vi "Process.vi"(8 "error in":errorcluster, 11 "Edit.Funnel":refnum<class "Edit.Funnel.lvclass">) -> (0 "error out":errorcluster, 3 "Edit.Funnel out":refnum<class "Edit.Funnel.lvclass">)   [LabVIEW 2019, in "Edit.Funnel.lvclass"]
doc: "---------------------------------------------------------------\nJKI State Machine Objects™\nhttp://jki.net/state-machine-objects/\nCopyright (C) 2005-2015, JKI <info@jki.net>\nALL RIGHTS RESERVED"
uses:
  Edit.Funnel.lvclass
  C:/Program Files (x86)/National Instruments/LabVIEW 2019/vi.lib/JKI/JKI SMO/SMO/SMO.lvclass
  <vilib>/JKI/JKI SMO/SMO/Typedefs/Parent Call--Enum.ctl
  Settings/Funnel Settings/Funnel Settings.lvclass/Funnel Settings.ctl
  Settings/ObjectSettings/ObjectSettings.lvclass/ObjectSettings.ctl
  subVIs/typedefs/Schedule Types/Schedule--Constant.ctl
  Settings/Setting Database/Setting Database.lvclass
  Settings/Funnel Settings/Funnel Settings.lvclass
  C:/Users/Albro/Documents/GitHub/AFM-Lithography/lvsrc/Classes/Settings/ObjectSettings/ObjectSettings.lvclass
  <vilib>/Utility/miscctls.llb/LVPointTypeDef.ctl
  <vilib>/JKI/JKI SMO/SMO/SMO.lvclass/SMO.ctl
  Settings/Setting Database/Typedefs/PrivateEvents--Setting Database.Copy Settings To Group.ctl
  Settings/Setting Database/Typedefs/PrivateEvents--Setting Database.SetDefaultFunnel.ctl
  Settings/Setting Database/Typedefs/PrivateEvents--Setting Database.CopyActiveFunnelToAll.ctl
  Settings/Funnel Settings/Accessors/Write Bottom Segments.vi
  Settings/ObjectSettings/Accessors/Write Resistance.vi
  Settings/ObjectSettings/Accessors/Read Speed Settings.vi
  Settings/ObjectSettings/Accessors/Read Voltage Settings.vi
  Settings/ObjectSettings/Accessors/Write Enabled.vi
  Settings/ObjectSettings/Accessors/Write Voltage Schedule.vi
  Settings/ObjectSettings/Accessors/Write Speed Schedule.vi
  Settings/ObjectSettings/Accessors/Write Direction.vi
  Settings/Funnel Settings/Accessors/Write Smooth Segments.vi
  Settings/ObjectSettings/Accessors/Read Enabled.vi
  Settings/ObjectSettings/Accessors/Read Direction.vi
  Settings/Funnel Settings/Accessors/Read Smooth Segments.vi
  Settings/Funnel Settings/Accessors/Read Bottom Segments.vi
  Settings/ObjectSettings/Accessors/Read Speed Schedule.vi
  Settings/ObjectSettings/Accessors/Read Voltage Schedule.vi
  Settings/ObjectSettings/Accessors/Read Resistance.vi
  <vilib>/JKI/JKI SMO/SMO/Private/ReftoDVR--SMO.vi
  Edit/Edit.lvclass
  <vilib>/JKI/JKI SMO/SMO/SMO.lvclass
  Settings/ObjectSettings/ObjectSettings.lvclass
panel:
  in  "Apply":bool
  in  "Apply All":bool
  out "Group String":string
  out "ID String":string
  in  "Copy to All":bool
  in  "Smooth Segments":dbl caption="Numeric 2"
  in  "Direction":u16(ring) caption="Ring" items=["Forward", "Backward"]
  in  "Speed Schedule":u16(ring) caption="Ring" items=["Constant", "Ramp", "Fn. Generator", "Formula"]
  in  "Voltage Schedule":u16(ring) caption="Ring" items=["Constant", "Ramp", "Fn. Generator", "Formula"]
  in  "Speed Settings":bool
  in  "Voltage Settings":bool
  in  "Enabled?":bool=TRUE
  in  "Voltage (V)":dbl caption="Numeric 2"
  in  "Speed (um/s)":dbl caption="Numeric 2"
  in  "Set Resistance":T1(ring) caption="Enum"
  in  "Bottom Segments":dbl caption="Numeric 2"
  in  "Save Default":bool
  # "For instructions on how to use the JKI State Machine Objects, examples and video tutorials, visit:\nhttp://jki.net/state-machine-objects/\n\nJKI State Machine Objects™\nhttp://jki.net/state-machine-objects/\nCopyright (C) 2005-2015, JKI <info@jki.net>\nALL RIGHTS RESERVED"
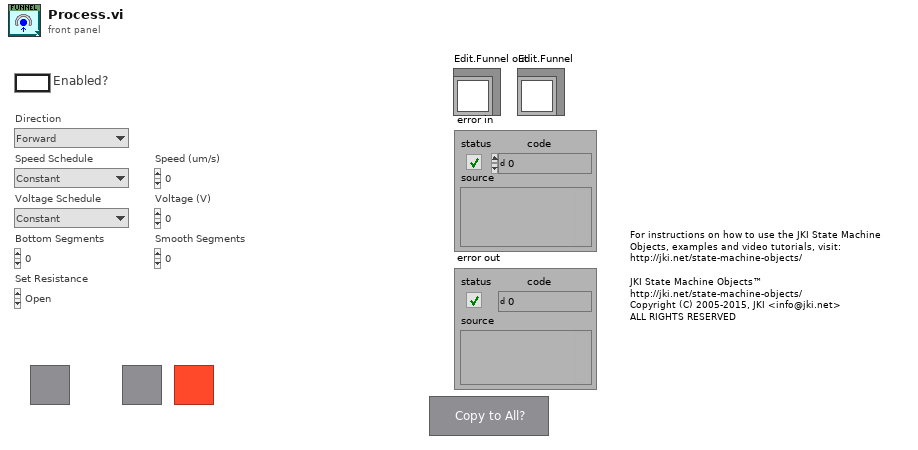
[diagram p1: front panel]
types:
  T1 = enum16{"Open", "Discharge Tip", "0 ohm", "100 kohm", "10 Mohm", "1 Gohm"}
  T2 = typedef "SMO.lvclass/Parent Call--Enum.ctl" = enum16{"Allows parent to run", "Does not request parent to run"}
  T3 = typedef "Schedule--Constant.ctl" = cluster{"Value":dbl}
  T4 = enum32{"invalid app kind", "Development System", "Run Time System", "Student Edition", "Embedded LabVIEW", "Evaluation", "Custom"}
  T5 = typedef "LVPointTypeDef.ctl" = cluster{"Horizontal":i16, "Vertical":i16}
  T6 = enum8{"Enabled", "Disabled", "Disabled and Grayed Out"}
  T7 = enum32{"Invalid", "Standard", "Closed", "Hidden", "Minimized", "Maximized"}
  T8 = enum32{"Bad", "Idle", "Run top level", "Running"}
  T9 = typedef "Setting Database.lvclass/PrivateEvents--Setting Database.Copy Settings To Group.ctl" = cluster{"Name":string, "Group":string}
  T10 = typedef "Setting Database.lvclass/PrivateEvents--Setting Database.SetDefaultFunnel.ctl" = bool
  T11 = typedef "Setting Database.lvclass/PrivateEvents--Setting Database.CopyActiveFunnelToAll.ctl" = bool
  T12 = typedef "Setting Database.lvclass/PublicEvents--Setting Database.NewActiveFunnel.ctl" = refnum<class "Funnel Settings.lvclass">
  T13 = cluster{"Core":cluster{"Current VI Reference":refnum<vi>, "Close Panel on Exit?":bool, "error":errorcluster}, "Self":refnum<class "Edit.Funnel.lvclass">, "SettingDB":refnum<class "Setting Database.lvclass">, "Funnel Settings":refnum<class "Funnel Settings.lvclass">}
  T14 = cluster{"Current VI Reference":refnum<vi>, "Close Panel on Exit?":bool, "error":errorcluster}
  T15 = enum16{"Always On", "Always Off", "Off While Running"}
  T16 = typedef "SMO.lvclass/Protected Events.ctl" = cluster{"StopProcesses":refnum<user-event>, "AbortProcesses":refnum<user-event>, "Config Changed":refnum<user-event>, "Dependency":refnum<user-event>}
  T17 = typedef "Setting Database.lvclass/PublicEvents--Cluster.ctl" = cluster{"NewActivePath":refnum<user-event>, "PathsUpdated":refnum<user-event>, "RectanglesUpdated":refnum<user-event>, "NewActiveRectangle":refnum<user-event>, "NewActiveFunnel":refnum<user-event>, "FunnelsUpdated":refnum<user-event>, "NewActiveDot":refnum<user-event>, "DotsUpdated":refnum<user-event>}
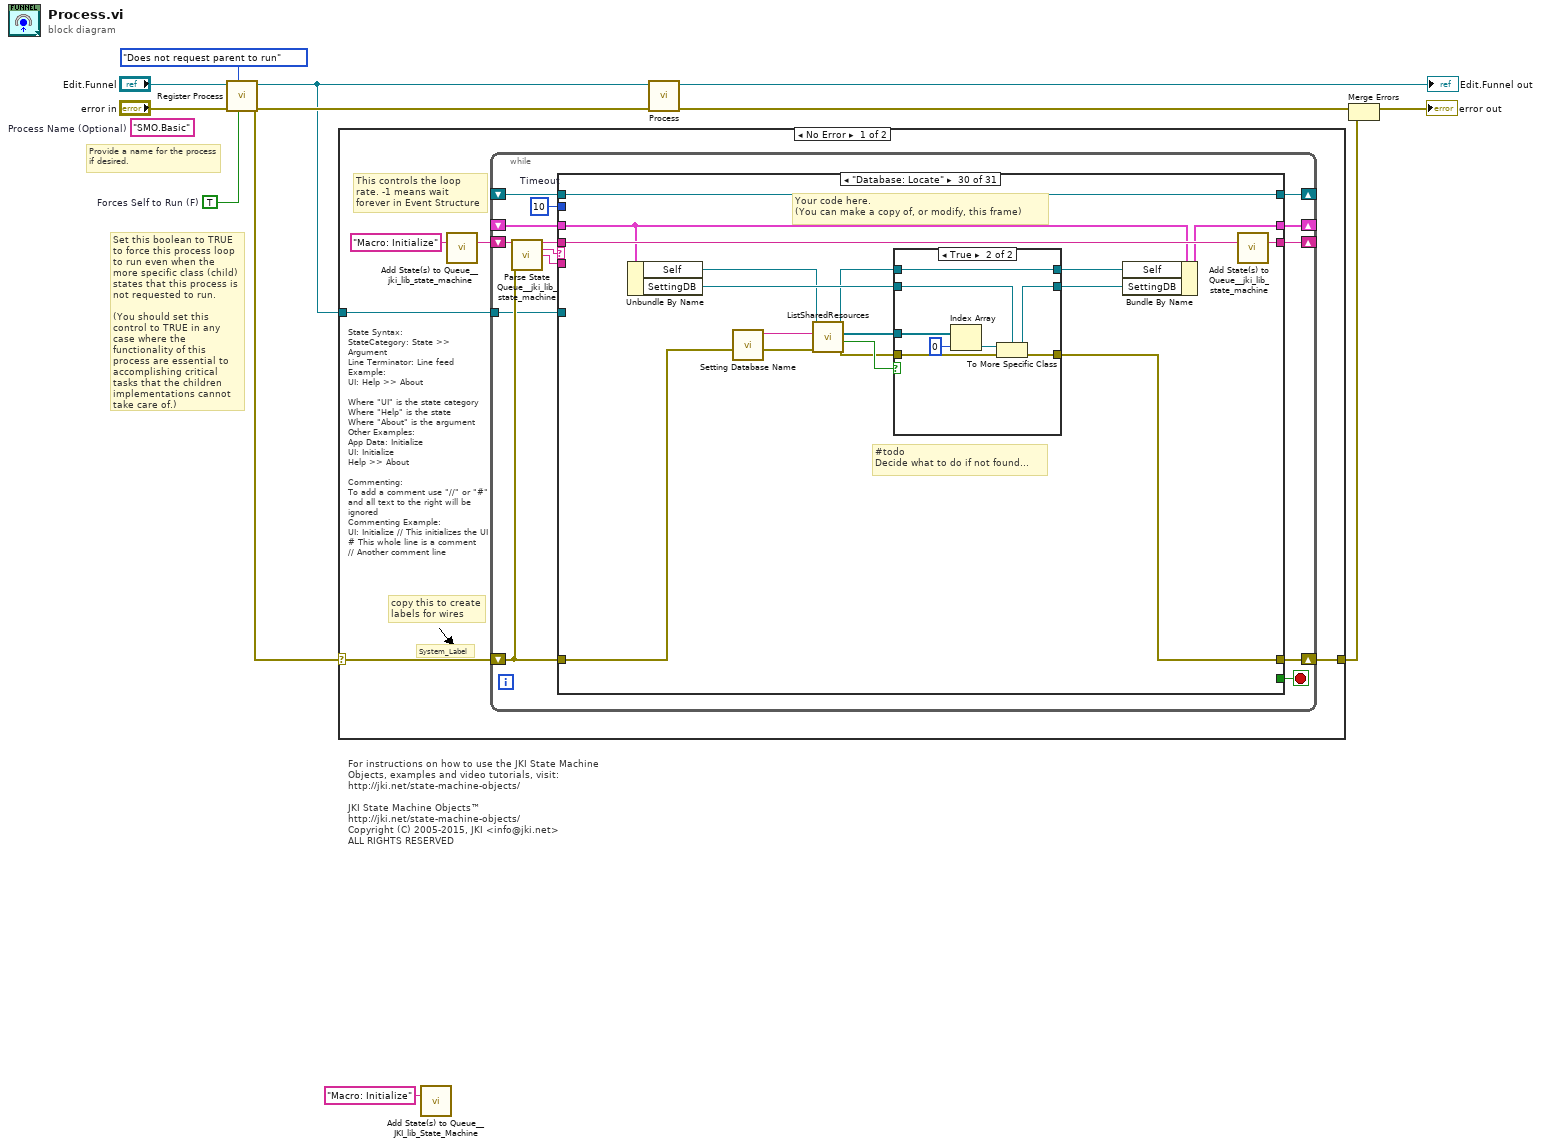
[diagram p0: block diagram]
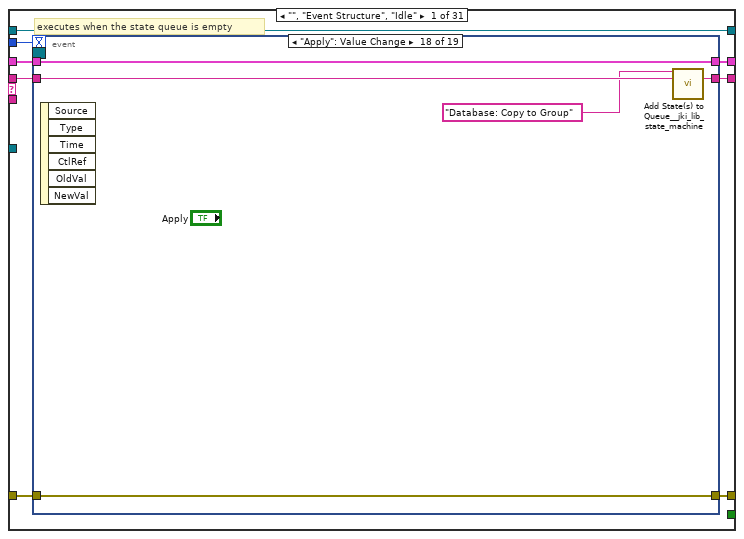
[diagram p2: hidden frame]
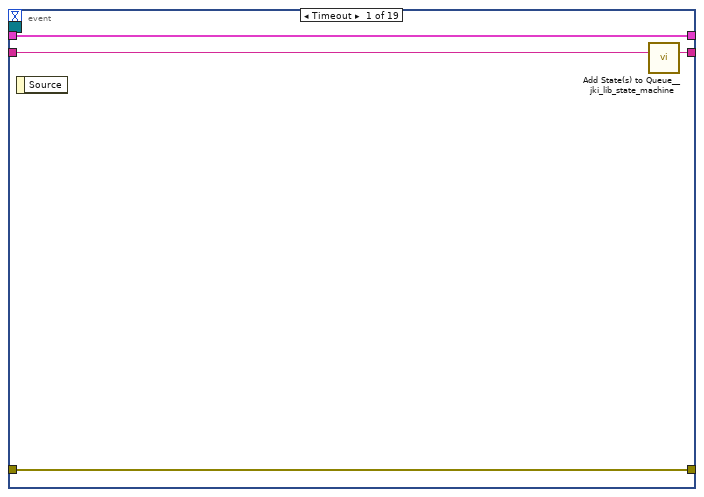
[diagram p3: hidden frame]
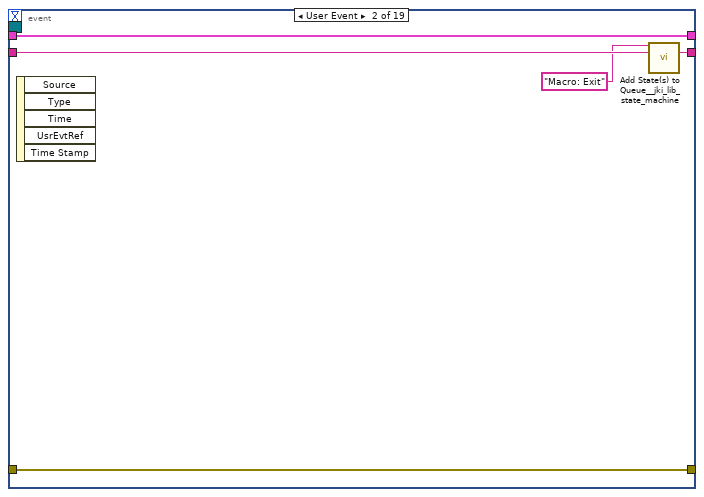
[diagram p4: hidden frame]
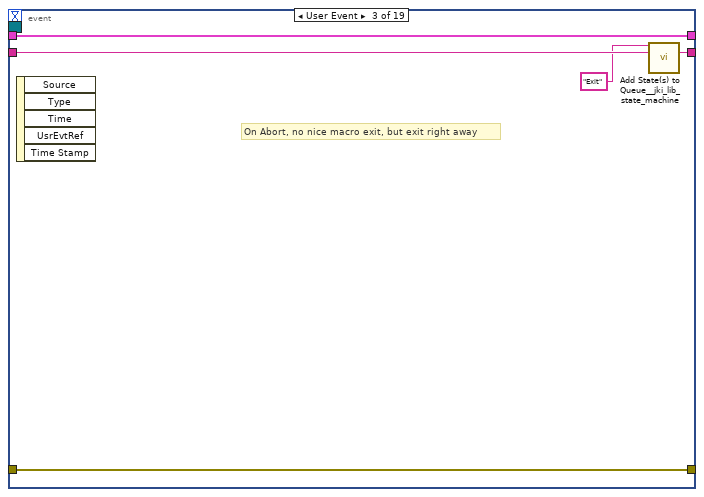
[diagram p5: hidden frame]
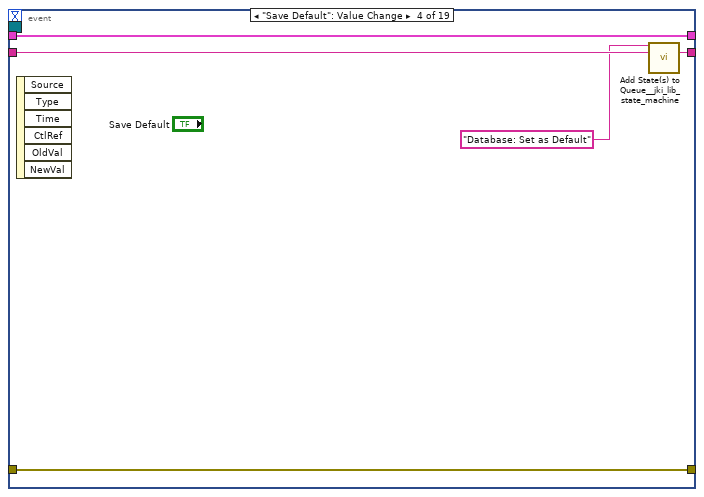
[diagram p6: hidden frame]
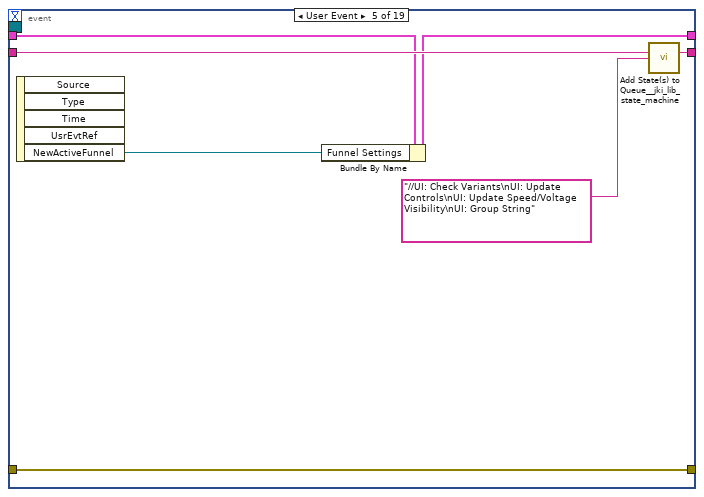
[diagram p7: hidden frame]
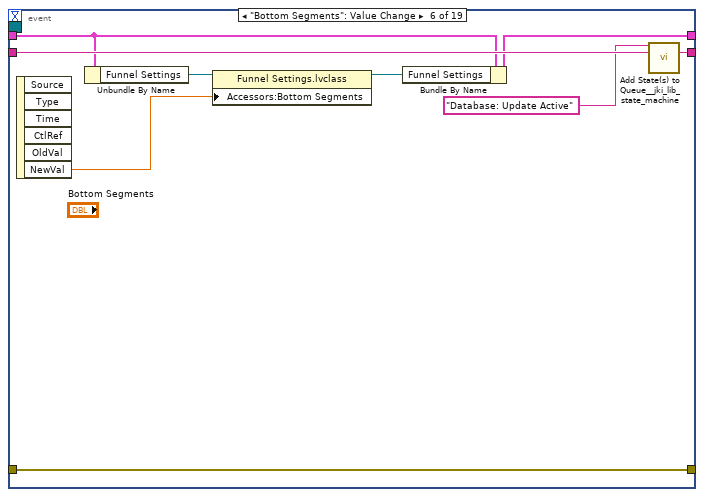
[diagram p8: hidden frame]
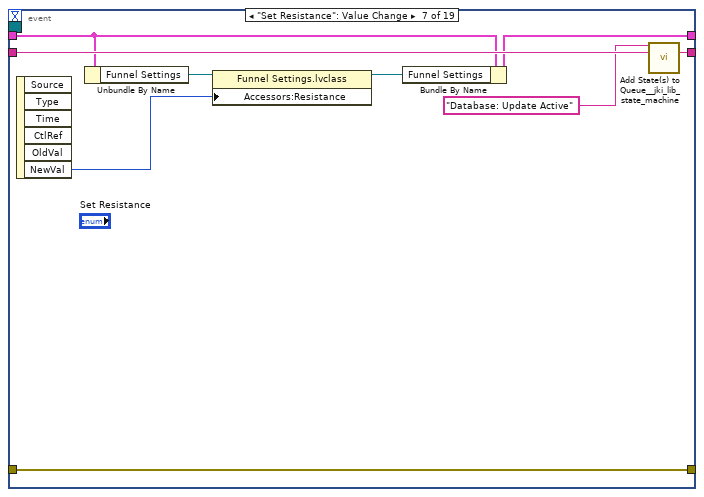
[diagram p9: hidden frame]
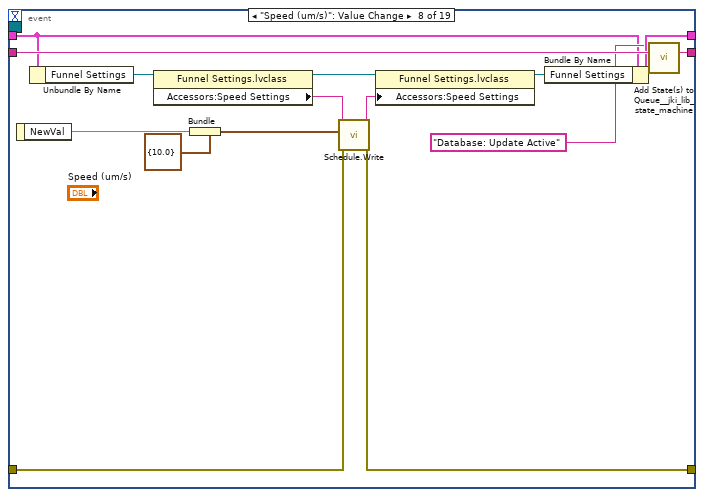
[diagram p10: hidden frame]
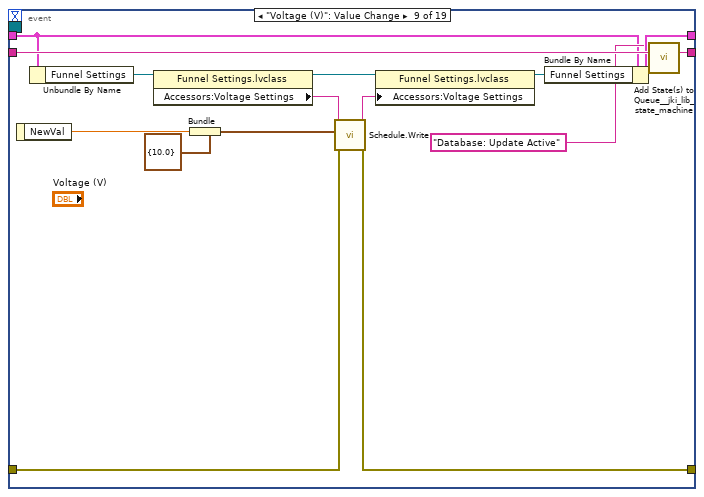
[diagram p11: hidden frame]
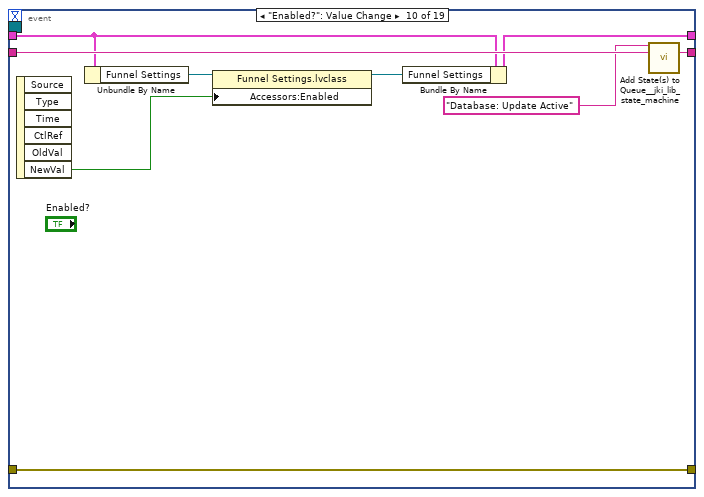
[diagram p12: hidden frame]
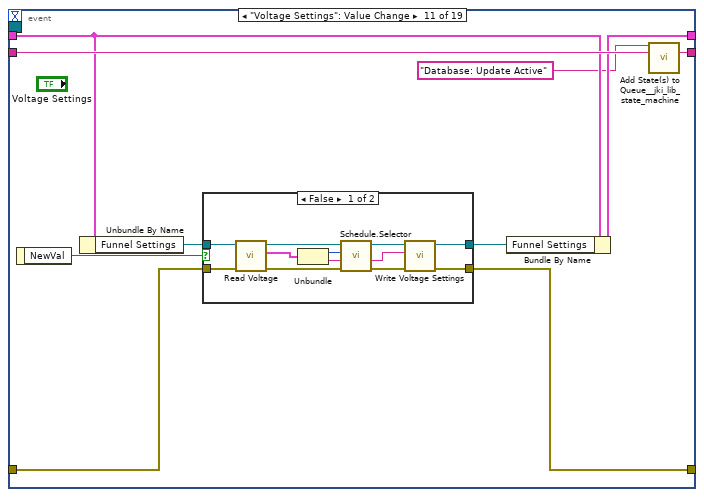
[diagram p13: hidden frame]
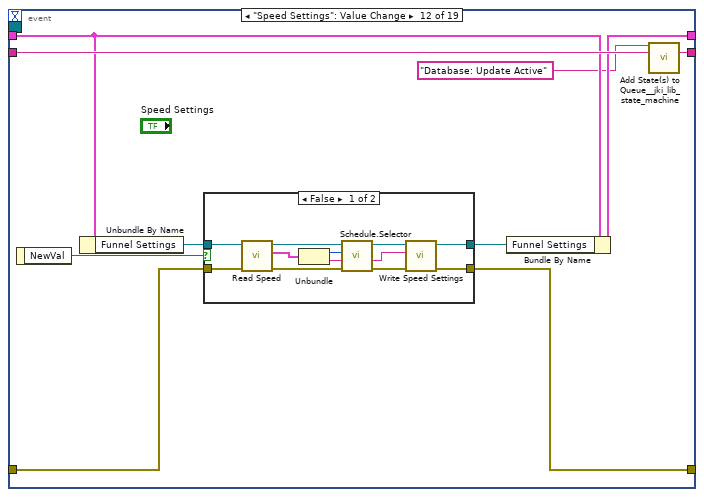
[diagram p15: hidden frame]
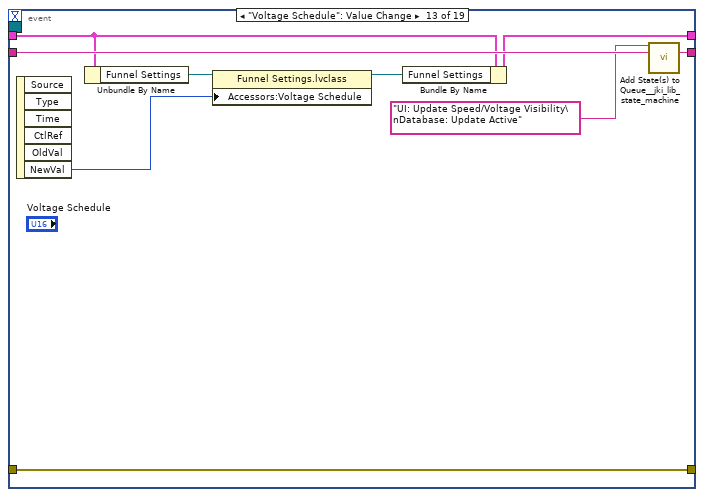
[diagram p17: hidden frame]
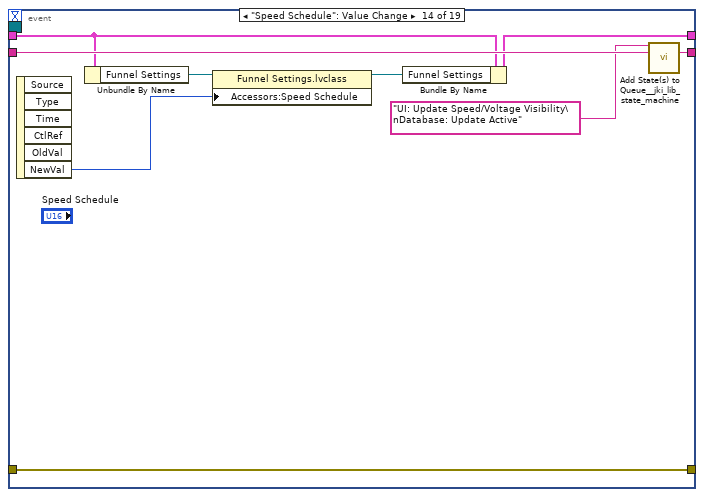
[diagram p18: hidden frame]
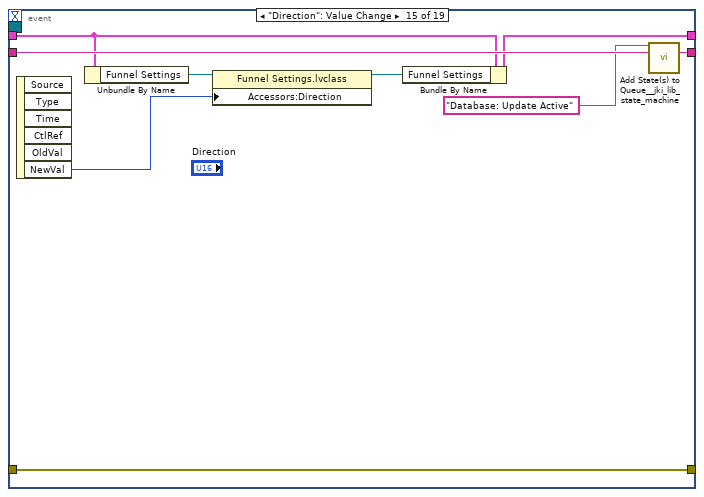
[diagram p19: hidden frame]
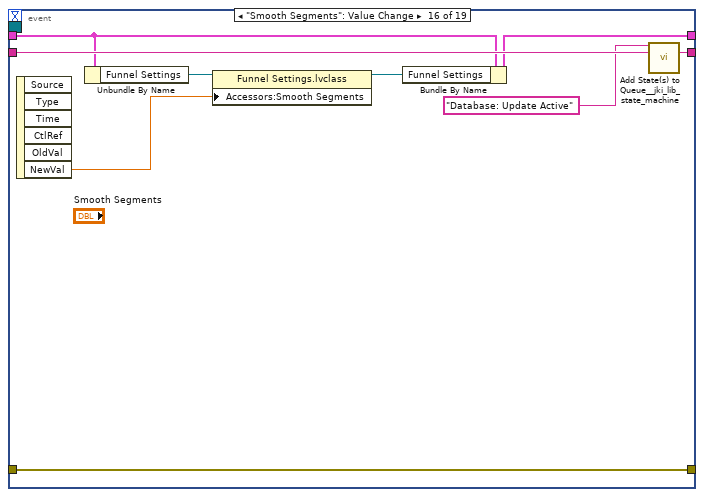
[diagram p20: hidden frame]
diagram:
  w3 = TRUE  # Forces Self to Run (F)
  (unwired) "SMO.Basic"  # Process Name (Optional)
  # "Provide a name for the process\nif desired."
  # "Set this boolean to TRUE to force this process loop to run even when the more specific class (child) states that this process is not requested to run.\n\n(You should set this control to TRUE in any case where the functionality of this process are essential to accomplishing critical tasks that the children implementations cannot take care of.)"
  # "For instructions on how to use the JKI State Machine Objects, examples and video tutorials, visit:\nhttp://jki.net/state-machine-objects/\n\nJKI State Machine Objects™\nhttp://jki.net/state-machine-objects/\nCopyright (C) 2005-2015, JKI <info@jki.net>\nALL RIGHTS RESERVED"
  n1 = call <vilib>:"Register Process.vi"("Forces Self to Run (F)"=w3, "Parent Call"=Parent_Call--Enum."Does not request parent to run", "error in (no error)"="error in", "SMO"="Edit.Funnel") -> ("error out"=w8:errorcluster, "SMO out"=w1:refnum<class "Edit.Funnel.lvclass">)  [unwired: 6 in]
  n2 = case shown="No Error" w8 {
    selector: w8 -> [w14 w583]
    tunnel: w1 -> [w13 _]
    tunnel: [w12 w583] -> w5
    frame No Error {
      # "State Syntax:\nStateCategory: State >> Argument\nLine Terminator: Line feed\nExample:\nUI: Help >> About\n\nWhere \"UI\" is the state category\nWhere \"Help\" is the state\nWhere \"About\" is the argument\nOther Examples:\nApp Data: Initialize\nUI: Initialize\nHelp >> About\n\nCommenting:\nTo add a comment use \"//\" or \"#\" and all text to the right will be ignored\nCommenting Example:\nUI: Initialize // This initializes the UI\n# This whole line is a comment\n// Another comment line"
      # "copy this to create labels for wires"
      # "This controls the loop rate. -1 means wait forever in Event Structure"
      # "System_Label"
      n3 = call <vilib>:"Add State(s) to Queue__jki_lib_state_machine.vi"("State(s) in (\"\")"="Macro: Initialize") -> ("States Out"=w15:string)  [unwired: 14 in]
      n4 = while "JKI - String-Based Queued State Machine (Basic) v1.0" {
        shift-right: [w23] -> _
        shift-left: _ -> [w22]
        shift-right: [w26] -> w12
        shift-left: w14 -> [w20]
        shift-right: [w25] -> _
        shift-left: w15 -> [w27]
        shift-right: [w19] -> _
        shift-left: _ -> [w18]
        tunnel: w13 -> [w17]
        stop <- w24 stop-if-true
        w21 = 10  # Timeout
        n5 = call <vilib>:"Parse State Queue__jki_lib_state_machine.vi"("State Queue"=w27, "Error In (no error)"=w20) -> ("Remaining States"=w29:string, "Current State"=w30:string, "Arguments"=w28:string)  [unwired: 11 in]
        n6 = case shown="\"Database: Locate\"" w30 {
          selector: w30 -> [_ _ w232 _ _ _ _ _ _ _ _ _ _ _ _ _ _ _ _ _ _ _ _ _ _ _ _ _ _ _ _]
          tunnel: w29 -> [w38 w226 w230 w251 w265 w271 w276 w288 w295 w300 w313 w327 w351 w366 w373 w392 w404 w436 w450 w464 w469 w480 w485 w498 w504 w509 w524 w534 w544 w561 w582]
          tunnel: w28 -> [_ _ _ _ _ _ _ _ _ _ _ _ _ _ w369 _ w399 _ _ _ _ _ _ _ _ _ _ _ _ _ _]
          tunnel: w22 -> [w36 w223 w231 w244 w252 w267 w273 _ w292 w297 w303 w320 w345 w358 w368 w390 w400 w433 w447 w451 w466 w473 w482 w494 w502 w506 w514 w526 w540 w548 w578]
          tunnel: [w35 w224 w235 w249 errorcluster {"status"=FALSE, "code"=0, "source"=""} ("error out") w266 w274 w280 w290 w298 w305 w322 w349 w363 w370 w379 w397 w434 w448 w462 w467 w471 w483 w493 w500 w507 w512 w529 w536 w546 w575] -> w26
          tunnel: w20 -> [w34 w224 w234 w249 w259 _ w274 w279 w291 w298 w307 w321 w349 w362 w371 w389 w398 w434 w448 w462 w467 w470 w483 w492 w500 w507 w511 w528 w537 w545 w574]
          tunnel: [w37 w225 w233 w250 w264 w270 w275 w287 w294 w299 w312 w326 w350 w365 w372 w391 w403 w435 w449 w463 w468 w479 w484 w497 w503 w508 w523 w533 w543 w560 w581] -> w25
          tunnel: [_ _ _ _ _ TRUE _ _ _ _ _ _ _ _ _ _ _ _ _ _ _ _ _ _ _ _ _ _ _ _ _] -> w24
          tunnel: [w33 w223 w231 w243 w258 w267 w273 w286 w292 w297 w303 w320 w345 w359 w368 w390 w400 w433 w447 w451 w466 w473 w482 w494 w502 w506 w515 w527 w541 w547 w579] -> w23
          tunnel: w21 -> [w32 _ _ _ _ _ _ _ _ _ _ _ _ _ _ _ _ _ _ _ _ _ _ _ _ _ _ _ _ _ _]
          tunnel: [w31 w222 w227 w239 w262 w268 w272 w284 w289 w296 w311 w325 w346 w361 w367 w378 w402 w432 w446 w461 w465 w478 w481 w496 w501 w505 w522 w532 w542 w559 w580] -> w19
          tunnel: w18 -> [w31 w222 w227 w239 w262 w268 w272 w284 w289 w296 w311 w325 w346 w361 w367 w378 w402 w432 w446 w461 w465 w478 w481 _ w501 w505 w522 w532 w542 w559 w580]
          tunnel: w17 -> [_ _ _ _ _ _ _ w282 _ _ _ _ _ _ _ _ _ _ _ _ _ _ _ _ _ _ _ _ _ _ _]
          frame "", "Event Structure", "Idle" {
            # "executes when the state queue is empty"
            n7 = event shown="[17] \"Apply\": Value Change" {
              selector: w31 -> [_ _ _ _ _ _ _ _ _ _ _ _ _ _ _ _ _ _ _]
              dyn-events: _ -> [_ _ _ _ _ _ _ _ _ _ _ _ _ _ _ _ _ _ _]
              timeout: w32 -> [_ _ _ _ _ _ _ _ _ _ _ _ _ _ _ _ _ _ _]
              tunnel: w38 -> [w42 w47 w52 w57 w64 w73 w82 w97 w112 w121 w131 w155 w178 w187 w196 w205 w210 w215 w221]
              tunnel: [w41 w46 w51 w56 w63 w72 w81 w96 w111 w120 w130 w154 w177 w186 w195 w204 w209 w214 w220] -> w37
              tunnel: w36 -> [w39 w44 w49 w54 w59 w69 w78 w90 w105 w117 w128 w152 w174 w183 w192 w201 w208 w213 w218]
              tunnel: [w40 w45 w50 w55 w62 w71 w80 w83 w98 w119 w124 w147 w176 w185 w194 w203 w207 w212 w219] -> w35
              tunnel: w34 -> [w40 w45 w50 w55 w62 w71 w80 w84 w99 w119 w123 w148 w176 w185 w194 w203 w207 w212 w219]
              tunnel: [w39 w44 w49 w54 w60 w70 w79 w95 w110 w118 w129 w153 w175 w184 w193 w202 w208 w213 w218] -> w33
              event Timeout {
                n8 = event-data() -> ()  [unwired: 1 in, 1 out]
                n9 = call <vilib>:"Add State(s) to Queue__jki_lib_state_machine.vi"("State(s) in (\"\")"=w42) -> ("States Out"=w41:string)  [unwired: 14 in]
              }
              event User Event {
                n10 = event-data() -> ()  [unwired: 1 in, 5 out]
                n11 = call <vilib>:"Add State(s) to Queue__jki_lib_state_machine.vi"("State(s) in Front (\"\")"="Macro: Exit" ("State(s) in Front (\"\")"), "State(s) in (\"\")"=w47) -> ("States Out"=w46:string)  [unwired: 13 in]
              }
              event User Event {
                # "On Abort, no nice macro exit, but exit right away"
                n12 = event-data() -> ()  [unwired: 1 in, 5 out]
                n13 = call <vilib>:"Add State(s) to Queue__jki_lib_state_machine.vi"("State(s) in Front (\"\")"="Exit" ("State(s) in Front (\"\")"), "State(s) in (\"\")"=w52) -> ("States Out"=w51:string)  [unwired: 13 in]
              }
              event "Save Default": Value Change {
                n14 = event-data() -> ()  [unwired: 1 in, 6 out]
                n15 = call <vilib>:"Add State(s) to Queue__jki_lib_state_machine.vi"("State(s) in Front (\"\")"="Database: Set as Default", "State(s) in (\"\")"=w57) -> ("States Out"=w56:string)  [unwired: 13 in]
              }
              event User Event {
                n16 = event-data() -> ("NewActiveFunnel"=w58:T12)  [unwired: 1 in, 4 out]
                n17 = Bundle By Name(cluster=w59, "Funnel Settings"=w58) -> (w60:T13)
                n18 = call <vilib>:"Add State(s) to Queue__jki_lib_state_machine.vi"("State(s) in (\"\")"=w64, "State(s) at Back (\"\")"="//UI: Check Variants\nUI: Update Controls\nUI: Update Speed/Voltage Visibility\nUI: Group String") -> ("States Out"=w63:string)  [unwired: 13 in]
              }
              event "Bottom Segments": Value Change {
                n19 = event-data() -> ("NewVal"=w66:dbl)  [unwired: 1 in, 5 out]
                n20 = Unbundle By Name(w69) -> ("Funnel Settings"=w68:refnum<class "Funnel Settings.lvclass">)
                n21 = property class="Funnel Settings.lvclass"(reference=w68, "Accessors:Bottom Segments"=w66) -> (reference out=w67:refnum<class "Funnel Settings.lvclass">)  [unwired: 1 in, 1 out]
                n22 = Bundle By Name(cluster=w69, "Funnel Settings"=w67) -> (w70:T13)
                n23 = call <vilib>:"Add State(s) to Queue__jki_lib_state_machine.vi"("State(s) in Front (\"\")"="Database: Update Active", "State(s) in (\"\")"=w73) -> ("States Out"=w72:string)  [unwired: 13 in]
              }
              event "Set Resistance": Value Change {
                n24 = event-data() -> ("NewVal"=w75:T1)  [unwired: 1 in, 5 out]
                n25 = Unbundle By Name(w78) -> ("Funnel Settings"=w77:refnum<class "Funnel Settings.lvclass">)
                n26 = property class="Funnel Settings.lvclass"(reference=w77, "Accessors:Resistance"=w75) -> (reference out=w76:refnum<class "Funnel Settings.lvclass">)  [unwired: 1 in, 1 out]
                n27 = Bundle By Name(cluster=w78, "Funnel Settings"=w76) -> (w79:T13)
                n28 = call <vilib>:"Add State(s) to Queue__jki_lib_state_machine.vi"("State(s) in Front (\"\")"="Database: Update Active", "State(s) in (\"\")"=w82) -> ("States Out"=w81:string)  [unwired: 13 in]
              }
              event "Speed (um/s)": Value Change {
                n29 = event-data() -> ("NewVal"=w88:dbl)  [unwired: 1 in]
                n30 = Unbundle By Name(w90) -> ("Funnel Settings"=w94:refnum<class "Funnel Settings.lvclass">)
                n31 = property class="Funnel Settings.lvclass"(reference=w94) -> (reference out=w93:refnum<class "Funnel Settings.lvclass">, "Accessors:Speed Settings"=w87:string)  [unwired: 1 in, 1 out]
                n32 = Bundle(cluster=T3 {"Value"=10.0} ("Constant"), "Value"=w88) -> (w85:T3)
                n33 = call "Schedule.Write.vi"("error in (no error)"=w84, "Data to Write"=w85, "Schedule <JSON> In"=w87) -> ("error out"=w83:errorcluster, "Schedule <JSON> Out"=w86:string)  [unwired: 7 in]
                n34 = property class="Funnel Settings.lvclass"(reference=w93, "Accessors:Speed Settings"=w86) -> (reference out=w91:refnum<class "Funnel Settings.lvclass">)  [unwired: 1 in, 1 out]
                n35 = Bundle By Name(cluster=w90, "Funnel Settings"=w91) -> (w95:T13)
                n36 = call <vilib>:"Add State(s) to Queue__jki_lib_state_machine.vi"("State(s) in Front (\"\")"="Database: Update Active", "State(s) in (\"\")"=w97) -> ("States Out"=w96:string)  [unwired: 13 in]
              }
              event "Voltage (V)": Value Change {
                n37 = event-data() -> ("NewVal"=w103:dbl)  [unwired: 1 in]
                n38 = Unbundle By Name(w105) -> ("Funnel Settings"=w109:refnum<class "Funnel Settings.lvclass">)
                n39 = property class="Funnel Settings.lvclass"(reference=w109) -> (reference out=w108:refnum<class "Funnel Settings.lvclass">, "Accessors:Voltage Settings"=w102:string)  [unwired: 1 in, 1 out]
                n40 = Bundle(cluster=T3 {"Value"=10.0} ("Constant"), "Value"=w103) -> (w100:T3)
                n41 = call "Schedule.Write.vi"("error in (no error)"=w99, "Data to Write"=w100, "Schedule <JSON> In"=w102) -> ("error out"=w98:errorcluster, "Schedule <JSON> Out"=w101:string)  [unwired: 7 in]
                n42 = property class="Funnel Settings.lvclass"(reference=w108, "Accessors:Voltage Settings"=w101) -> (reference out=w106:refnum<class "Funnel Settings.lvclass">)  [unwired: 1 in, 1 out]
                n43 = Bundle By Name(cluster=w105, "Funnel Settings"=w106) -> (w110:T13)
                n44 = call <vilib>:"Add State(s) to Queue__jki_lib_state_machine.vi"("State(s) in Front (\"\")"="Database: Update Active", "State(s) in (\"\")"=w112) -> ("States Out"=w111:string)  [unwired: 13 in]
              }
              event "Enabled?": Value Change {
                n45 = event-data() -> ("NewVal"=w114:bool)  [unwired: 1 in, 5 out]
                n46 = Unbundle By Name(w117) -> ("Funnel Settings"=w116:refnum<class "Funnel Settings.lvclass">)
                n47 = property class="Funnel Settings.lvclass"(reference=w116, "Accessors:Enabled"=w114) -> (reference out=w115:refnum<class "Funnel Settings.lvclass">)  [unwired: 1 in, 1 out]
                n48 = Bundle By Name(cluster=w117, "Funnel Settings"=w115) -> (w118:T13)
                n49 = call <vilib>:"Add State(s) to Queue__jki_lib_state_machine.vi"("State(s) in Front (\"\")"="Database: Update Active", "State(s) in (\"\")"=w121) -> ("States Out"=w120:string)  [unwired: 13 in]
              }
              event "Voltage Settings": Value Change {
                n50 = event-data() -> ("NewVal"=w122:bool)  [unwired: 1 in]
                n51 = Unbundle By Name(w128) -> ("Funnel Settings"=w126:refnum<class "Funnel Settings.lvclass">)
                n52 = case shown="False" w122 {
                  tunnel: w126 -> [w143 w145]
                  tunnel: [w135 w145] -> w125
                  tunnel: w123 -> [w142 w144]
                  tunnel: [w132 w144] -> w124
                  frame False {
                    n53 = call "Read Voltage.vi"("error in (no error)"=w142, "ObjectSettings in"=w143) -> ("error out"=w140:errorcluster, "Voltage"=w139:cluster{"Schedule":u16, "Settings":string}, "ObjectSettings out"=w141:refnum<class "Funnel Settings.lvclass">)  [unwired: 7 in]
                    n54 = Unbundle(w139) -> ("Schedule"=w138:u16, "Settings"=w137:string)
                    n55 = call-dynamic "Schedule.Selector.vi"("error in (no error)"=w140, "Settings In"=w137, "Schedule"=w138, "ObjectSettings in"=w141) -> ("error out"=w134:errorcluster, "Settings Out"=w133:string, "ObjectSettings out"=w136:refnum<class "Funnel Settings.lvclass">)  [unwired: 5 in]
                    n56 = call "Write Voltage Settings.vi"("error in (no error)"=w134, "Settings"=w133, "ObjectSettings in"=w136) -> ("error out"=w132:errorcluster, "ObjectSettings out"=w135:refnum<class "Funnel Settings.lvclass">)  [unwired: 7 in]
                  }
                  frame True {
                  }
                }
                n57 = Bundle By Name(cluster=w128, "Funnel Settings"=w125) -> (w129:T13)
                n58 = call <vilib>:"Add State(s) to Queue__jki_lib_state_machine.vi"("State(s) in Front (\"\")"="Database: Update Active", "State(s) in (\"\")"=w131) -> ("States Out"=w130:string)  [unwired: 13 in]
              }
              event "Speed Settings": Value Change {
                n59 = event-data() -> ("NewVal"=w149:bool)  [unwired: 1 in]
                n60 = Unbundle By Name(w152) -> ("Funnel Settings"=w150:refnum<class "Funnel Settings.lvclass">)
                n61 = case shown="False" w149 {
                  tunnel: w150 -> [w165 w169]
                  tunnel: [w159 w169] -> w146
                  tunnel: w148 -> [w163 w168]
                  tunnel: [w158 w168] -> w147
                  frame False {
                    n62 = call "Read Speed.vi"("error in (no error)"=w163, "ObjectSettings in"=w165) -> ("error out"=w162:errorcluster, "Speed"=w161:cluster{"Schedule":u16, "Settings":string}, "ObjectSettings out"=w164:refnum<class "Funnel Settings.lvclass">)  [unwired: 7 in]
                    n63 = Unbundle(w161) -> ("Schedule"=w167:u16, "Settings"=w166:string)
                    n64 = call-dynamic "Schedule.Selector.vi"("error in (no error)"=w162, "Settings In"=w166, "Schedule"=w167, "ObjectSettings in"=w164) -> ("error out"=w157:errorcluster, "Settings Out"=w156:string, "ObjectSettings out"=w160:refnum<class "Funnel Settings.lvclass">)  [unwired: 5 in]
                    n65 = call "Write Speed Settings.vi"("error in (no error)"=w157, "Settings"=w156, "ObjectSettings in"=w160) -> ("error out"=w158:errorcluster, "ObjectSettings out"=w159:refnum<class "Funnel Settings.lvclass">)  [unwired: 7 in]
                  }
                  frame True {
                  }
                }
                n66 = Bundle By Name(cluster=w152, "Funnel Settings"=w146) -> (w153:T13)
                n67 = call <vilib>:"Add State(s) to Queue__jki_lib_state_machine.vi"("State(s) in Front (\"\")"="Database: Update Active", "State(s) in (\"\")"=w155) -> ("States Out"=w154:string)  [unwired: 13 in]
              }
              event "Voltage Schedule": Value Change {
                n68 = event-data() -> ("NewVal"=w171:u16)  [unwired: 1 in, 5 out]
                n69 = Unbundle By Name(w174) -> ("Funnel Settings"=w173:refnum<class "Funnel Settings.lvclass">)
                n70 = property class="Funnel Settings.lvclass"(reference=w173, "Accessors:Voltage Schedule"=w171) -> (reference out=w172:refnum<class "Funnel Settings.lvclass">)  [unwired: 1 in, 1 out]
                n71 = Bundle By Name(cluster=w174, "Funnel Settings"=w172) -> (w175:T13)
                n72 = call <vilib>:"Add State(s) to Queue__jki_lib_state_machine.vi"("State(s) in Front (\"\")"="UI: Update Speed/Voltage Visibility\nDatabase: Update Active", "State(s) in (\"\")"=w178) -> ("States Out"=w177:string)  [unwired: 13 in]
              }
              event "Speed Schedule": Value Change {
                n73 = event-data() -> ("NewVal"=w180:u16)  [unwired: 1 in, 5 out]
                n74 = Unbundle By Name(w183) -> ("Funnel Settings"=w182:refnum<class "Funnel Settings.lvclass">)
                n75 = property class="Funnel Settings.lvclass"(reference=w182, "Accessors:Speed Schedule"=w180) -> (reference out=w181:refnum<class "Funnel Settings.lvclass">)  [unwired: 1 in, 1 out]
                n76 = Bundle By Name(cluster=w183, "Funnel Settings"=w181) -> (w184:T13)
                n77 = call <vilib>:"Add State(s) to Queue__jki_lib_state_machine.vi"("State(s) in Front (\"\")"="UI: Update Speed/Voltage Visibility\nDatabase: Update Active", "State(s) in (\"\")"=w187) -> ("States Out"=w186:string)  [unwired: 13 in]
              }
              event "Direction": Value Change {
                n78 = event-data() -> ("NewVal"=w189:u16)  [unwired: 1 in, 5 out]
                n79 = Unbundle By Name(w192) -> ("Funnel Settings"=w191:refnum<class "Funnel Settings.lvclass">)
                n80 = property class="Funnel Settings.lvclass"(reference=w191, "Accessors:Direction"=w189) -> (reference out=w190:refnum<class "Funnel Settings.lvclass">)  [unwired: 1 in, 1 out]
                n81 = Bundle By Name(cluster=w192, "Funnel Settings"=w190) -> (w193:T13)
                n82 = call <vilib>:"Add State(s) to Queue__jki_lib_state_machine.vi"("State(s) in Front (\"\")"="Database: Update Active", "State(s) in (\"\")"=w196) -> ("States Out"=w195:string)  [unwired: 13 in]
              }
              event "Smooth Segments": Value Change {
                n83 = event-data() -> ("NewVal"=w198:dbl)  [unwired: 1 in, 5 out]
                n84 = Unbundle By Name(w201) -> ("Funnel Settings"=w200:refnum<class "Funnel Settings.lvclass">)
                n85 = property class="Funnel Settings.lvclass"(reference=w200, "Accessors:Smooth Segments"=w198) -> (reference out=w199:refnum<class "Funnel Settings.lvclass">)  [unwired: 1 in, 1 out]
                n86 = Bundle By Name(cluster=w201, "Funnel Settings"=w199) -> (w202:T13)
                n87 = call <vilib>:"Add State(s) to Queue__jki_lib_state_machine.vi"("State(s) in Front (\"\")"="Database: Update Active", "State(s) in (\"\")"=w205) -> ("States Out"=w204:string)  [unwired: 13 in]
              }
              event "Copy to All", "Apply All": Value Change {
                n88 = event-data() -> ()  [unwired: 1 in, 6 out]
                n89 = call <vilib>:"Add State(s) to Queue__jki_lib_state_machine.vi"("State(s) in Front (\"\")"="Database: Copy to All", "State(s) in (\"\")"=w210) -> ("States Out"=w209:string)  [unwired: 13 in]
              }
              event "Apply": Value Change {
                n90 = event-data() -> ()  [unwired: 1 in, 6 out]
                n91 = call <vilib>:"Add State(s) to Queue__jki_lib_state_machine.vi"("State(s) in Front (\"\")"="Database: Copy to Group", "State(s) in (\"\")"=w215) -> ("States Out"=w214:string)  [unwired: 13 in]
              }
              event Panel Close? {
                # "Discard the event because we'll close the front panel ourselves in Macro: Exit"
                # "Close Panel button (pressed) Event\n(this executes Macro: Exit to terminate the VI)"
                n92 = event-data() -> ()  [unwired: 1 in, 1 out]
                n93 = event-data("Discard?"=TRUE) -> ()  [unwired: 1 in, 1 out]
                n94 = call <vilib>:"Add State(s) to Queue__jki_lib_state_machine.vi"("State(s) in Front (\"\")"="Macro: Exit", "State(s) in (\"\")"=w221) -> ("States Out"=w220:string)  [unwired: 13 in]
              }
            }
          }
          frame "---------- Core ----------" {
            # "Do not put any code in this frame.\n(it is a separator no-op)"
            n95 = call <vilib>:"Add State(s) to Queue__jki_lib_state_machine.vi"("State(s) in (\"\")"=w226) -> ("States Out"=w225:string)  [unwired: 14 in]
          }
          frame Default {
            w238 = 42 items=["No error", "Argument error", "Memory is full", "Out of zone", "End of file", "File already open", "Generic file I/O error", "File not found", "File permission error", "Disk is full", "Duplicate path", "Too many files open", "System feature not enabled", "Resource file not found", "Cannot add resource", "Resource not found", "Image not found", "Image memory error", "Pen does not exist", "Config type invalid", "Config token not found", "Config parse error", "Config memory error", "Bad external code format", "Bad external code offset", "External code not present", "Null window", "Destroy window error", "Null menu", "Print aborted", "Bad print record", "Print driver error", "Windows error during printing", "Memory error during printing", "Print dialog error", "Generic print error", "Invalid device refnum", "Device not found", "Device parameter error", "Device unit error", "Cannot open device", "Device call aborted", "Generic error", "Cancelled by user", "Object ID too low", "Object ID too high", "Object not in heap", "Unknown heap", "Unknown object (invalid DefProc)", "Unknown object (DefProc not in table)", "Message out of range", "Invalid (null) method", "Unknown message", "Manager call not supported", "Bad address", "Network operation in progress", "Network operation timed out", "Connection is busy", "Network attribute not supported", "Network error", "Address in use", "System out of memory", "Connection aborted", "Connection refused", "Not connected", "Already connected", "Connection closed", "Initialization error (interapplication manager)", "Bad occurrence", "Wait on unbound occurrence handler", "Occurrence queue overflow", "Datalog type conflict", "Unused", "Unrecognized type (interapplication manager)", "Memory corrupt", "Failed to make temporary DLL", "Old CIN version", "Drag socket not found", "Failed to load drop-object", "Failed to register OLE object", "Failed to release OLE object", "Format specifier type mismatch", "Unknown format specifier", "Too few format specifiers", "Too many format specifiers", "Scan failed", "Newer CIN version", "Error converting to variant", "Runtime menu error", "Password tampered", "Variant attribute not found", "Incompatible variant data type", "Event data is not available", "Event Store is not present", "Occurrence is not found", "Event Queue is not created", "Event info is not available", "Refnum passed is NULL", "Error retrieving Class GUID", "Error retrieving CoClass GUID", "Error retrieving TypeLib GUID.", "Bad built application magic bytes.", "Specific driver is different from the specific driver associated with the Logical Name.", "There is no session opened to the class driver.", "Max Error", "MAX - Error with config objects", "MAX - Error loading configuration", "MAX - Group not supported"]
            # "Current State"
            # "Do not delete, rename, or modify this frame.\n(this is used to capture unhandled states and typos)"
            # "Handle mistyped state name (developer tool)"
            n96 = Format Into String(format string="Software Exception: Unhandled State \"%s\"." ("message"), error in=w234, w232) -> (resulting string=w237:string, error out=w236:errorcluster)  [unwired: 1 in]
            n97 = call <vilib>:"Error Cluster From Error Code.vi"("show call chain? (False)"=TRUE, "error in (no error)"=w236, "error message (\"\")"=w237, "error code (0)"=w238) -> ("error out"=w235:errorcluster)  [unwired: 5 in]
            n98 = call <vilib>:"Add State(s) to Queue__jki_lib_state_machine.vi"("State(s) in (\"\")"=w230) -> ("States Out"=w233:string)  [unwired: 14 in]
          }
          frame "Initialize Core Data" {
            # "exe?"
            # "If panel starts closed or is an EXE, then close it when we exit"
            # "Do not delete, rename, or modify this frame.\n(this is used to determine panel behavior on exit)"
            n99 = control-ref of="Current VI Reference"() -> (w248:refnum<vi>)
            n100 = property class="VI"() -> ("Front Panel.Open"=w247:bool)  [unwired: 2 in, 2 out]
            n101 = property class="App"() -> ("App.Kind"=w246:T4)  [unwired: 2 in, 2 out]
            n102 = Not(x=w247) -> (.not. x?=w242:bool)
            n103 = Equal?(x=w246, y=T4."Run Time System" ("Application:Kind")) -> (x = y?=w241:bool)
            n104 = Or(x=w242, y=w241) -> (x .or. y?=w245:bool)
            n105 = Bundle By Name(cluster=w244, "Core.Current VI Reference"=w248, "Core.Close Panel on Exit?"=w245) -> (w243:T13)
            n106 = call <vilib>:"Add State(s) to Queue__jki_lib_state_machine.vi"("State(s) in (\"\")"=w251) -> ("States Out"=w250:string)  [unwired: 14 in]
          }
          frame "Error Handler" {
            w261 = TRUE  # Stop on Unhandled Error (T)
            # "Handle any errors here.\nYou can also output any states to clean-up after errors occur"
            # "Clear error"
            n107 = Unbundle By Name(w252) -> ("Self"=w260:refnum<class "Edit.Funnel.lvclass">)
            n108 = call-dynamic "Handle Error.vi"("Stop on Unhandled Error (T)"=w261, "error in"=w259, "SMO"=w260) -> ("handling error"=w254:errorcluster, "Unhandled error"=w257:errorcluster)  [unwired: 6 in, 1 out]
            n109 = Bundle By Name(cluster=w252, "Core.error"=w257) -> (w258:T13)
            n110 = Select(t="Exit", s=w254, f="") -> (s? t:f=w253:string)
            n111 = call <vilib>:"Add State(s) to Queue__jki_lib_state_machine.vi"("State(s) in Front (\"\")"=w253, "State(s) in (\"\")"=w265) -> ("States Out"=w264:string)  [unwired: 13 in]
          }
          frame "Exit" {
            # "Do not put any code in this frame.\n(No errors that occur here will be handled.)"
            n112 = Unbundle By Name(w267) -> ("Core.error"=w266:errorcluster)
            n113 = call <vilib>:"Add State(s) to Queue__jki_lib_state_machine.vi"("State(s) in (\"\")"=w271) -> ("States Out"=w270:string)  [unwired: 14 in]
          }
          frame "---------- Data ----------" {
            # "Do not put any code in this frame.\n(It is a separator no-op. You can make a copy of this frame to create a new Data frame)"
            n114 = call <vilib>:"Add State(s) to Queue__jki_lib_state_machine.vi"("State(s) in (\"\")"=w276) -> ("States Out"=w275:string)  [unwired: 14 in]
          }
          frame "Data: Initialize" {
            w281 = refnum<class "Edit.Funnel.lvclass"> refnum  # Self
            w283 = refnum<class "Funnel Settings.lvclass"> refnum  # Funnel Settings
            w278 = refnum<class "Setting Database.lvclass"> refnum  # SettingDB
            w285 = T14 {"Current VI Reference"=refnum, "Close Panel on Exit?"=FALSE, "error"={"status"=FALSE, "code"=0, "source"=""}}  # Core
            # "Initialize the shift-register data, here.\n(data names are defined by what you wire into the bundle function)"
            n115 = Variant To Data(error in=w279, type=w281, Variant=w282) -> (data=w277:refnum<class "Edit.Funnel.lvclass">, error out=w280:errorcluster)
            n116 = Bundle("Core"=w285, "Self"=w277, "SettingDB"=w278, "Funnel Settings"=w283) -> (w286:T13)  [unwired: 1 in]
            n117 = call <vilib>:"Add State(s) to Queue__jki_lib_state_machine.vi"("State(s) in (\"\")"=w288) -> ("States Out"=w287:string)  [unwired: 14 in]
          }
          frame "Data: Cleanup" {
            # "Cleanup any data and references, here.\n(this is called automatically, by the Macro: Exit)"
            n118 = Unbundle By Name(w292) -> ("Core.Current VI Reference"=w293:refnum<vi>)
            n119 = Close Reference(reference=w293, error in (no error)=w291) -> (error out=w290:errorcluster)
            n120 = call <vilib>:"Add State(s) to Queue__jki_lib_state_machine.vi"("State(s) in (\"\")"=w295) -> ("States Out"=w294:string)  [unwired: 14 in]
          }
          frame "---------- UI ----------" {
            # "Do not put any code in this frame.\n(It is a separator no-op. You can make a copy of this frame to create a new UI frame)"
            n121 = call <vilib>:"Add State(s) to Queue__jki_lib_state_machine.vi"("State(s) in (\"\")"=w300) -> ("States Out"=w299:string)  [unwired: 14 in]
          }
          frame "UI: Group String" {
            # "Do not put any code in this frame.\n(It is a separator no-op. You can make a copy of this frame to create a new UI frame)"
            n122 = Unbundle By Name(w303) -> ("Funnel Settings"=w308:refnum<class "Funnel Settings.lvclass">)
            n123 = control-ref of="Apply"() -> (w304:refnum<vi>)
            n124 = call-dynamic "Read GUID.vi"("ObjectSettings in"=w308) -> ("GUID"=→"ID String":string)  [unwired: 8 in, 2 out]
            n125 = call-dynamic "Read Group.vi"("error in (no error)"=w307, "ObjectSettings in"=w308) -> ("error out"=w306:errorcluster, "Group"=w301:string)  [unwired: 7 in, 1 out]
            "Group String" <- w301
            n126 = Empty String/Path?(string/path=w301) -> (empty?=w310:bool)
            n127 = Not(x=w310) -> (.not. x?=w309:bool)
            n128 = property class="Bool"(reference=w304, error in=w306, "Visible"=w309) -> (error out=w305:errorcluster)  [unwired: 1 out]
            n129 = call <vilib>:"Add State(s) to Queue__jki_lib_state_machine.vi"("State(s) in (\"\")"=w313) -> ("States Out"=w312:string)  [unwired: 14 in]
          }
          frame "UI: Initialize" {
            w315 = T15."Off While Running" ("Horizontal Scrollbar Visibility")
            # "Initialize the User Interface, here.\n(this is called automatically, by the Macro: Init)"
            n130 = Unbundle By Name(w320) -> ("Core.Current VI Reference"=w319:refnum<vi>)
            n131 = control-ref of="Speed Schedule"() -> (w324:refnum<vi>)
            n132 = property class="Ring (strict)"(reference=w324, error in=w321, "DisabledEnum"=T6."Disabled and Grayed Out" ("Disabled")) -> (error out=w322:errorcluster)  [unwired: 1 out]
            n133 = property class="VI"(reference=w319) -> ("Panel"=w318:refnum<vi>)  [unwired: 1 in, 2 out]
            n134 = property class="Pnl"(reference=w318) -> ("Panes[]"=w317:refnum<vi>[])  [unwired: 1 in, 2 out]
            n135 = Index Array(array=w317) -> (element=w316:refnum<vi>)  [unwired: 1 in]
            n136 = property class="Pane"(reference=w316, "HorizScrollbarVisibility"=w315, "VertScrollbarVisibility"=w315, "Origin"=T5 {"Horizontal"=0, "Vertical"=0}) -> ()  [unwired: 1 in, 2 out]
            n137 = call <vilib>:"Add State(s) to Queue__jki_lib_state_machine.vi"("State(s) in (\"\")"=w327) -> ("States Out"=w326:string)  [unwired: 14 in]
          }
          frame "UI: Update Controls" {
            w332 = T3 {"Value"=10.0} ("Constant")
            # "Using Variant Attr. For Settings"
            n138 = Unbundle By Name(w345) -> ("Funnel Settings"=w338:refnum<class "Funnel Settings.lvclass">)
            n139 = property class="Funnel Settings.lvclass"(reference=w338) -> ("Accessors:Enabled"=w344:bool, "Accessors:Direction"=w343:u16, "Accessors:Smooth Segments"=w342:dbl, "Accessors:Bottom Segments"=w341:dbl, "Accessors:Speed Schedule"=w340:u16, "Accessors:Voltage Schedule"=w339:u16, "Accessors:Resistance"=w337:T1, "Accessors:Speed Settings"=w330:string, "Accessors:Voltage Settings"=w328:string)  [unwired: 1 in, 2 out]
            n140 = local write "Direction"(w343) -> ()
            n141 = local write "Bottom Segments"(w341) -> ()
            n142 = local write "Voltage Schedule"(w339) -> ()
            n143 = call "Schedule.CheckVariantAttributes.vi"("Schedule <JSON> In"=w330) -> ("Schedule <JSON> Out"=w331:string)  [unwired: 9 in, 1 out]
            n144 = call "Schedule.CheckVariantAttributes.vi"("Schedule <JSON> In"=w328) -> ("Schedule <JSON> Out"=w329:string)  [unwired: 9 in, 1 out]
            n145 = call "Schedule.Read.vi"("Data to Read"=w332, "Schedule <JSON> In"=w331) -> ("Data Out"=w336:variant)  [unwired: 7 in, 2 out]
            n146 = call "Schedule.Read.vi"("Data to Read"=w332, "Schedule <JSON> In"=w329) -> ("Data Out"=w335:variant)  [unwired: 7 in, 2 out]
            n147 = local write "Enabled?"(w344) -> ()
            n148 = local write "Smooth Segments"(w342) -> ()
            n149 = local write "Speed Schedule"(w340) -> ()
            n150 = local write "Set Resistance"(w337) -> ()
            n151 = Variant To Data(type=w332, Variant=w336) -> (data=w333:T3)  [unwired: 1 in, 1 out]
            n152 = Variant To Data(type=w332, Variant=w335) -> (data=w334:T3)  [unwired: 1 in, 1 out]
            n153 = Unbundle(w334) -> ("Value"=w347:dbl)
            n154 = Unbundle(w333) -> ("Value"=w348:dbl)
            n155 = local write "Speed (um/s)"(w348) -> ()
            n156 = local write "Voltage (V)"(w347) -> ()
            n157 = call <vilib>:"Add State(s) to Queue__jki_lib_state_machine.vi"("State(s) in (\"\")"=w351) -> ("States Out"=w350:string)  [unwired: 14 in]
          }
          frame "UI: Check Variants" {
            # "Do not put any code in this frame.\n(It is a separator no-op. You can make a copy of this frame to create a new UI frame)"
            n158 = Unbundle By Name(w358) -> ("Funnel Settings"=w360:refnum<class "Funnel Settings.lvclass">)
            n159 = property class="Funnel Settings.lvclass"(reference=w360) -> (reference out=w356:refnum<class "Funnel Settings.lvclass">, "Accessors:Speed Settings"=w355:string, "Accessors:Voltage Settings"=w352:string)  [unwired: 1 in, 1 out]
            n160 = call "Schedule.CheckVariantAttributes.vi"("error in (no error)"=w362, "Schedule <JSON> In"=w355) -> ("error out"=w364:errorcluster, "Schedule <JSON> Out"=w354:string)  [unwired: 8 in]
            n161 = call "Schedule.CheckVariantAttributes.vi"("error in (no error)"=w364, "Schedule <JSON> In"=w352) -> ("error out"=w363:errorcluster, "Schedule <JSON> Out"=w353:string)  [unwired: 8 in]
            n162 = property class="Funnel Settings.lvclass"(reference=w356, "Accessors:Speed Settings"=w354, "Accessors:Voltage Settings"=w353) -> (reference out=w357:refnum<class "Funnel Settings.lvclass">)  [unwired: 1 in, 1 out]
            n163 = Bundle By Name(cluster=w358, "Funnel Settings"=w357) -> (w359:T13)
            n164 = call <vilib>:"Add State(s) to Queue__jki_lib_state_machine.vi"("State(s) in (\"\")"=w366) -> ("States Out"=w365:string)  [unwired: 14 in]
          }
          frame "UI: Cursor Set" {
            # "Argument"
            # "Set and Unset Cursor Busy.\n(Usage: \"UI: Cursor Set >> Busy|Idle\")"
            n165 = case shown="\"Idle\", Default" w369 {
              tunnel: w371 -> [w375 w377]
              tunnel: [w374 w376] -> w370
              frame "Idle", Default {
                n166 = call <vilib>:"Unset Busy.vi"("error in (no error)"=w375) -> ("error out"=w374:errorcluster)  [unwired: 10 in]
              }
              frame "Busy" {
                n167 = call <vilib>:"Set Busy.vi"("error in (no error)"=w377) -> ("error out"=w376:errorcluster)  [unwired: 9 in, 1 out]
              }
            }
            n168 = call <vilib>:"Add State(s) to Queue__jki_lib_state_machine.vi"("State(s) in (\"\")"=w373) -> ("States Out"=w372:string)  [unwired: 14 in]
          }
          frame "UI: Update Speed/Voltage Visibility" {
            n169 = local read "Voltage Schedule"() -> (w386:u16)
            n170 = local read "Speed Schedule"() -> (w385:u16)
            n171 = case shown="0" w386 {
              tunnel: [TRUE FALSE] -> w388
              frame 0 {
              }
              frame 1, Default {
              }
            }
            n172 = case shown="0" w385 {
              tunnel: [TRUE FALSE] -> w387
              frame 0 {
              }
              frame 1, Default {
              }
            }
            n173 = property on="Voltage (V)" class="DigNum (strict)"(error in=w389, "Visible"=w388) -> (error out=w384:errorcluster)  [unwired: 1 in, 1 out]
            n174 = Not(x=w388) -> (.not. x?=w382:bool)
            n175 = property on="Voltage Settings" class="Bool (strict)"(error in=w384, "Visible"=w382) -> (error out=w383:errorcluster)  [unwired: 1 in, 1 out]
            n176 = property on="Speed (um/s)" class="DigNum (strict)"(error in=w383, "Visible"=w387) -> (error out=w381:errorcluster)  [unwired: 1 in, 1 out]
            n177 = Not(x=w387) -> (.not. x?=w380:bool)
            n178 = property on="Speed Settings" class="Bool (strict)"(error in=w381, "Visible"=w380) -> (error out=w379:errorcluster)  [unwired: 1 in, 1 out]
            n179 = call <vilib>:"Add State(s) to Queue__jki_lib_state_machine.vi"("State(s) in (\"\")"=w392) -> ("States Out"=w391:string)  [unwired: 14 in]
          }
          frame "UI: Front Panel State" {
            # "Argument"
            # "Set Front Panel Open or Closed\n(Usage: \"UI: Front Panel State >> Open|Close\")"
            n180 = Unbundle By Name(w400) -> ("Core.Current VI Reference"=w401:refnum<vi>)
            n181 = disable-structure shown="Default" {
              disable-tunnel: w398 -> [w408 w431]
              disable-tunnel: [w407 w431] -> w397
              disable-tunnel: w401 -> [w406 _]
              disable-tunnel: w399 -> [w405 _]
              frame condition #0 (active) {
                n182 = case shown="\"Close\"" w405 {
                  tunnel: w408 -> [w412 w425]
                  tunnel: [w414 w426] -> w407
                  tunnel: w406 -> [w413 w423]
                  frame "Open", Default {
                    n183 = property class="VI"(reference=w413, error in=w412) -> (reference out=w410:refnum<vi>, error out=w411:errorcluster, "FP.State"=w409:T7)
                    n184 = case shown="\"Closed\"" w409 {
                      tunnel: [w417 w420] -> w414
                      tunnel: w411 -> [w416 w420]
                      tunnel: w410 -> [w415 _]
                      frame "Closed" {
                        n185 = invoke class="VI" method="FP.Open"(reference=w415, error in=w416, "Activate"=TRUE, "State"=T7."Standard") -> (error out=w417:errorcluster)  [unwired: 1 in, 4 out]
                      }
                      frame Default {
                      }
                    }
                  }
                  frame "Close" {
                    n186 = property class="VI"(reference=w423, error in=w425) -> (reference out=w422:refnum<vi>, error out=w424:errorcluster, "FP.State"=w421:T7)
                    n187 = case shown="Default" w421 {
                      tunnel: [w427 w430] -> w426
                      tunnel: w424 -> [w427 w429]
                      tunnel: w422 -> [_ w428]
                      frame "Invalid", "Closed" {
                      }
                      frame Default {
                        n188 = invoke class="VI" method="FP.Close"(reference=w428, error in=w429) -> (error out=w430:errorcluster)  [unwired: 1 in, 2 out]
                      }
                    }
                  }
                }
              }
              frame condition #1 {
              }
            }
            n189 = call <vilib>:"Add State(s) to Queue__jki_lib_state_machine.vi"("State(s) in (\"\")"=w404) -> ("States Out"=w403:string)  [unwired: 14 in]
          }
          frame "---------- Macro ----------" {
            # "Do not put any code in this frame.\n(It is a separator no-op. You can make a copy of this frame to create a new Macro frame)"
            n190 = call <vilib>:"Add State(s) to Queue__jki_lib_state_machine.vi"("State(s) in (\"\")"=w436) -> ("States Out"=w435:string)  [unwired: 14 in]
          }
          frame "Macro: Initialize" {
            w441 = "UI: Initialize\n//UI: Front Panel State >> Open"  # UI: Initialize //UI: Front Panel State >> Open
            w438 = "Process: Sync"
            (unwired) "Data: Initialize\nInitialize Core Data\nDatabase: Locate\nEvents: Register\nUI: Initialize\n//UI: Check Variants\n//UI: Update Controls\n//UI: Update Speed/Voltage Visibility\nUI: Front Panel State >> Close"
            # "Initialization Macro\n(This is called once, when the VI starts)"
            n191 = control-ref of="This VI"() -> (w440:refnum<vi>)
            n192 = property class="VI"(reference=w440) -> ("Exec.State"=w439:T8)  [unwired: 1 in, 2 out]
            n193 = Equal?(x=w439, y=T8."Run top level") -> (x = y?=w444:bool)
            n194 = Select(t=w438, s=w444, f="") -> ()  [unwired: 1 out]
            n195 = call <vilib>:"Add State(s) to Queue__jki_lib_state_machine.vi"("State(s) in Front (\"\")"="Data: Initialize\nInitialize Core Data\nDatabase: Locate\nEvents: Register", "State(s) in (\"\")"=w438, "State(s) at Back (\"\")"=w441) -> ("States Out"=w437:string)  [unwired: 12 in]
            n196 = call <vilib>:"Add State(s) to Queue__jki_lib_state_machine.vi"("State(s) in Front (\"\")"=w437, "State(s) in (\"\")"=w450) -> ("States Out"=w449:string)  [unwired: 13 in]
          }
          frame "Macro: Exit" {
            # "Exit Macro\n(This is called once, when the VI exits)"
            n197 = Unbundle By Name(w451) -> ("Core.Close Panel on Exit?"=w460:bool)
            n198 = Select(t="UI: Front Panel State >> Close", s=w460, f="") -> (s? t:f=w457:string)
            n199 = call <vilib>:"Add State(s) to Queue__jki_lib_state_machine.vi"("State(s) in Front (\"\")"="Data: Cleanup\nEvents: Unregister", "State(s) in (\"\")"="Process: Sync", "State(s) at Back (\"\")"="Exit") -> ("States Out"=w454:string)  [unwired: 12 in]
            n200 = call <vilib>:"Add State(s) to Queue__jki_lib_state_machine.vi"("State(s) in (\"\")"=w457, "State(s) at Back (\"\")"=w454) -> ("States Out"=w452:string)  [unwired: 13 in]
            n201 = call <vilib>:"Add State(s) to Queue__jki_lib_state_machine.vi"("State(s) in Front (\"\")"=w452, "State(s) in (\"\")"=w464) -> ("States Out"=w463:string)  [unwired: 13 in]
          }
          frame "---------- Process ----------" {
            # "Do not put any code in this frame.\n(It is a separator no-op. You can make a copy of this frame to create a new Macro frame)"
            n202 = call <vilib>:"Add State(s) to Queue__jki_lib_state_machine.vi"("State(s) in (\"\")"=w469) -> ("States Out"=w468:string)  [unwired: 14 in]
          }
          frame "Process: Sync" {
            # "Do not put any code in this frame.\n(It is a separator no-op. You can make a copy of this frame to create a new Macro frame)"
            n203 = Unbundle By Name(w473) -> ("Self"=w474:refnum<class "Edit.Funnel.lvclass">)
            n204 = call <vilib>:"WaitOnProcessSync.vi"("error in (no error)"=w470, "SMO"=w474) -> ("error out"=w471:errorcluster, "Don't run?"=w477:bool)  [unwired: 7 in, 1 out]
            n205 = Select(t="Data: Cleanup\nEvents: Unregister\nExit", s=w477, f="") -> (s? t:f=w472:string)
            n206 = call <vilib>:"Add State(s) to Queue__jki_lib_state_machine.vi"("State(s) in Front (\"\")"=w472, "State(s) in (\"\")"=w480) -> ("States Out"=w479:string)  [unwired: 13 in]
          }
          frame "---------- Events ----------" {
            # "Do not put any code in this frame.\n(It is a separator no-op. You can make a copy of this frame to create a new UI frame)"
            n207 = call <vilib>:"Add State(s) to Queue__jki_lib_state_machine.vi"("State(s) in (\"\")"=w485) -> ("States Out"=w484:string)  [unwired: 14 in]
          }
          frame "Events: Register" {
            # "Do not put any code in this frame.\n(It is a separator no-op. You can make a copy of this frame to create a new UI frame)"
            n208 = Unbundle By Name(w494) -> ("SettingDB"=w490:refnum<class "Setting Database.lvclass">, "Self"=w488:refnum<class "Edit.Funnel.lvclass">)
            n209 = call <vilib>:"GetProtectedEvents.vi"("SMO"=w488) -> ("error out"=w486:errorcluster, "SMO Protected Events"=w487:T16)  [unwired: 8 in, 1 out]
            n210 = call "Setting Database.GetPublicEvents.vi"("Setting Database"=w490) -> ("error out"=w491:errorcluster, "Public Events"=w489:T17)  [unwired: 8 in, 1 out]
            n211 = register-events(w489, w487) -> (reference out=w496:refnum<event-registration>, error out=w495:errorcluster)  [unwired: 2 in]
            n212 = Merge Errors(w492, w495, w491, w486) -> (w493:errorcluster)
            n213 = call <vilib>:"Add State(s) to Queue__jki_lib_state_machine.vi"("State(s) in (\"\")"=w498) -> ("States Out"=w497:string)  [unwired: 14 in]
          }
          frame "Events: Unregister" {
            # "Do not put any code in this frame.\n(It is a separator no-op. You can make a copy of this frame to create a new UI frame)"
            n214 = Unregister For Events(event registration refnum=w501, error in=w500) -> (error out=w499:errorcluster)
            n215 = call <vilib>:"Clear Errors.vi"("error in (no error)"=w499) -> ()  [unwired: 5 in, 2 out]
            n216 = call <vilib>:"Add State(s) to Queue__jki_lib_state_machine.vi"("State(s) in (\"\")"=w504) -> ("States Out"=w503:string)  [unwired: 14 in]
          }
          frame "---------- Database ----------" {
            # "Template Separator\n(You can make a copy of, or modify, this frame)"
            n217 = call <vilib>:"Add State(s) to Queue__jki_lib_state_machine.vi"("State(s) in (\"\")"=w509) -> ("States Out"=w508:string)  [unwired: 14 in]
          }
          frame "Database: Copy to Group" {
            # "Template Separator\n(You can make a copy of, or modify, this frame)"
            n218 = Unbundle By Name(w514) -> ("SettingDB"=w520:refnum<class "Setting Database.lvclass">, "Funnel Settings"=w521:refnum<class "Funnel Settings.lvclass">)
            n219 = call-dynamic "Read Group.vi"("error in (no error)"=w511, "ObjectSettings in"=w521) -> ("error out"=w513:errorcluster, "Group"=w517:string)  [unwired: 7 in, 1 out]
            n220 = Bundle By Name(cluster=T9 {"Name"="", "Group"=""} ("Copy Settings To Group"), "Group"=w517, "Name"="f") -> (w516:T9)
            n221 = call "Setting Database.CopySettingsToGroup.vi"("error in (no error)"=w513, "Copy Settings To Group"=w516, "Setting Database"=w520) -> ("error out"=w512:errorcluster, "Setting Database out"=w518:refnum<class "Setting Database.lvclass">)  [unwired: 7 in]
            n222 = Bundle By Name(cluster=w514, "SettingDB"=w518) -> (w515:T13)
            n223 = call <vilib>:"Add State(s) to Queue__jki_lib_state_machine.vi"("State(s) in (\"\")"=w524) -> ("States Out"=w523:string)  [unwired: 14 in]
          }
          frame "Database: Set as Default" {
            # "Template Separator\n(You can make a copy of, or modify, this frame)"
            n224 = Unbundle By Name(w526) -> ("SettingDB"=w531:refnum<class "Setting Database.lvclass">)
            n225 = call "Setting Database.SetDefaultFunnel.vi"("error in (no error)"=w528, "SetDefaultFunnel"=T10 TRUE, "Setting Database"=w531) -> ("error out"=w529:errorcluster, "Setting Database out"=w525:refnum<class "Setting Database.lvclass">)  [unwired: 7 in]
            n226 = Bundle By Name(cluster=w526, "SettingDB"=w525) -> (w527:T13)
            n227 = call <vilib>:"Add State(s) to Queue__jki_lib_state_machine.vi"("State(s) in (\"\")"=w534) -> ("States Out"=w533:string)  [unwired: 14 in]
          }
          frame "Database: Copy to All" {
            # "Template Separator\n(You can make a copy of, or modify, this frame)"
            n228 = Unbundle By Name(w540) -> ("SettingDB"=w535:refnum<class "Setting Database.lvclass">)
            n229 = call "Setting Database.CopyActiveFunnelToAll.vi"("error in (no error)"=w537, "CopyActiveFunnelToAll"=T11 TRUE, "Setting Database"=w535) -> ("error out"=w536:errorcluster, "Setting Database out"=w539:refnum<class "Setting Database.lvclass">)  [unwired: 7 in]
            n230 = Bundle By Name(cluster=w540, "SettingDB"=w539) -> (w541:T13)
            n231 = call <vilib>:"Add State(s) to Queue__jki_lib_state_machine.vi"("State(s) in (\"\")"=w544) -> ("States Out"=w543:string)  [unwired: 14 in]
          }
          frame "Database: Locate" {
            # "#todo\nDecide what to do if not found..."
            # "Your code here.\n(You can make a copy of, or modify, this frame)"
            n232 = Unbundle By Name(w548) -> ("Self"=w553:refnum<class "Edit.Funnel.lvclass">, "SettingDB"=w556:refnum<class "Setting Database.lvclass">)
            n233 = call "Setting Database Name.vi"("error in (no error)"=w545) -> ("error out"=w550:errorcluster, "Name"=w549:string)  [unwired: 9 in]
            n234 = call <vilib>:"ListSharedResources.vi"("error in (no error)"=w550, "Filter (regex|name)"=w549, "SMO in"=w553) -> ("error out"=w551:errorcluster, "resources found?"=w554:bool, "Shared Resources"=w558:refnum<class "SMO.lvclass">[], "SMO out"=w552:refnum<class "Edit.Funnel.lvclass">)  [unwired: 5 in]
            n235 = case shown="True" w554 {
              tunnel: w558 -> [_ w572]
              tunnel: [w563 w568] -> w557
              tunnel: w556 -> [w563 w570]
              tunnel: w552 -> [w564 w569]
              tunnel: [w564 w569] -> w555
              tunnel: w551 -> [w562 w565]
              tunnel: [w562 w566] -> w546
              frame False {
              }
              frame True {
                n236 = Index Array(array=w572, index=0) -> (element=w571:refnum<class "SMO.lvclass">)
                n237 = To More Specific Class(target class=w570, reference=w571, error in=w565) -> (specific class reference=w568:refnum<class "Setting Database.lvclass">, error out=w566:errorcluster)
              }
            }
            n238 = Bundle By Name(cluster=w548, "Self"=w555, "SettingDB"=w557) -> (w547:T13)
            n239 = call <vilib>:"Add State(s) to Queue__jki_lib_state_machine.vi"("State(s) in (\"\")"=w561) -> ("States Out"=w560:string)  [unwired: 14 in]
          }
          frame "Database: Update Active" {
            # "Your code here.\n(You can make a copy of, or modify, this frame)"
            n240 = Unbundle By Name(w578) -> ("SettingDB"=w577:refnum<class "Setting Database.lvclass">, "Funnel Settings"=w573:refnum<class "Funnel Settings.lvclass">)
            n241 = call "Setting Database.UpdateActiveFunnel.vi"("error in (no error)"=w574, "UpdateActiveFunnel"=w573, "Setting Database"=w577) -> ("error out"=w575:errorcluster, "Setting Database"=w576:refnum<class "Setting Database.lvclass">)  [unwired: 7 in]
            n242 = Bundle By Name(cluster=w578, "SettingDB"=w576) -> (w579:T13)
            n243 = call <vilib>:"Add State(s) to Queue__jki_lib_state_machine.vi"("State(s) in (\"\")"=w582) -> ("States Out"=w581:string)  [unwired: 14 in]
          }
        }
      }
    }
    frame Error {
    }
  }
  n244 = call <vilib>:"Add State(s) to Queue__JKI_lib_State_Machine.vi"("State(s) in (\"\")"="Macro: Initialize") -> ()  [unwired: 14 in, 1 out]
  n245 = call-parent "Process.vi"("error in"=w8, "Edit"=w1) -> ("error out"=w6:errorcluster, "Edit out"=→"Edit.Funnel out":refnum<class "Edit.Funnel.lvclass">)  [unwired: 8 in]
  n246 = Merge Errors(w6, w5) -> (→"error out":errorcluster)
